vi "LSX Get Ctr Fast Move Counter.vi"(0 "lLSID":i32, 1 "plRC":i32, 5 "plXC":i32, 7 "plYC":i32, 9 "plZC":i32, 11 "error in (no error)":errorcluster) -> (3 "plRC out":i32, 4 "function return":i32, 6 "plXC out":i32, 8 "plYC out":i32, 10 "plZC out":i32, 15 "error out":errorcluster)   [LabVIEW 2016, in "Tango_DLL.lvlib"]
doc: "TANGOAPI int TANGOCALL LSX_GetCtrFastMoveCounter (int lLSID, int *plXC, int *plYC, int *plZC, int *plRC);"
uses:
  Tango_DLL.lvlib
  2017/Microscope Control/Device Library/Stages/Marzhauser/SCAN IM 120 x 80/Tango DLL VIs/Tango_DLL.dll
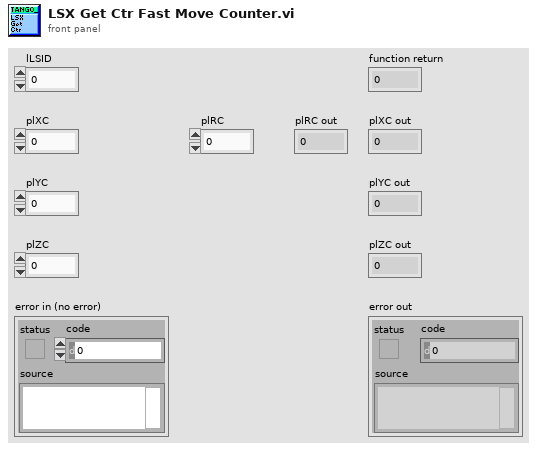
[diagram p1: front panel]
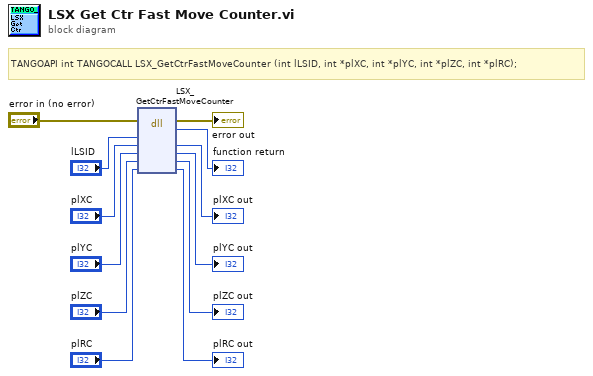
[diagram p0: block diagram]
diagram:
  # "TANGOAPI int TANGOCALL LSX_GetCtrFastMoveCounter (int lLSID, int *plXC, int *plYC, int *plZC, int *plRC);"
  n1 = dll-call lib="C:/Users/4PiSMS/Documents/Microscope Control/2017/Microscope Control/Device Library/Stages/Marzhauser/SCAN IM 120 x 80/Tango DLL VIs/Tango_DLL.*" fn="LSX_GetCtrFastMoveCounter"(error in="error in (no error)", "lLSID"="lLSID", "plXC"="plXC", "plYC"="plYC", "plZC"="plZC", "plRC"="plRC") -> (error out=→"error out":errorcluster, →"function return":i32, "plXC"=→"plXC out":i32, "plYC"=→"plYC out":i32, "plZC"=→"plZC out":i32, "plRC"=→"plRC out":i32)  [unwired: 3 in, 1 out]
